vi "pRACTICA_1Y2_Punto_2_4.vi"() -> ()   [LabVIEW 2020]
panel:
  in  "Enum":T1(ring)
  out "?":string="La division es:"
  out "?":dbl
  in  "Numero 2":dbl
  in  "Numero 1":dbl
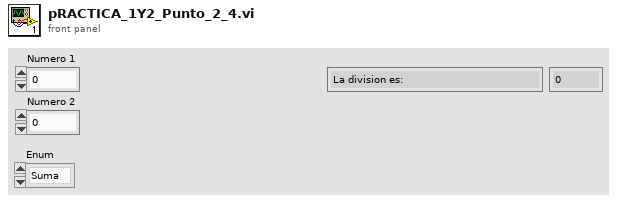
[diagram p1: front panel]
types:
  T1 = enum16{"Suma", "Resta", "Multiplicacion", "Division"}
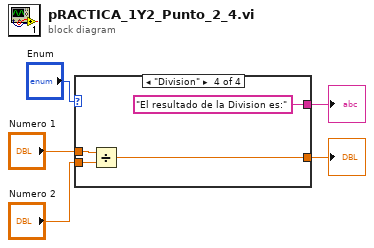
[diagram p0: block diagram]
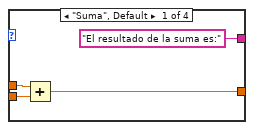
[diagram p2: hidden frame]
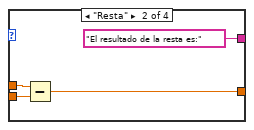
[diagram p3: hidden frame]
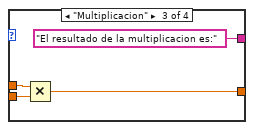
[diagram p4: hidden frame]
diagram:
  n1 = case shown="\"Division\"" "Enum" {
    tunnel: "Numero 1" -> [w9 w13 w16 w19]
    tunnel: "Numero 2" -> [w8 w12 w17 w20]
    tunnel: [w7 w11 w15 w18] -> w2
    tunnel: ["El resultado de la suma es:" "El resultado de la resta es:" "El resultado de la multiplicacion es:" "El resultado de la Division es:"] -> w1
    frame "Suma", Default {
      n2 = Add(x=w9, y=w8) -> (x+y=w7:dbl)
    }
    frame "Resta" {
      n3 = Subtract(x=w13, y=w12) -> (x-y=w11:dbl)
    }
    frame "Multiplicacion" {
      n4 = Multiply(x=w16, y=w17) -> (x*y=w15:dbl)
    }
    frame "Division" {
      n5 = Divide(x=w19, y=w20) -> (x/y=w18:dbl)
    }
  }
  "?" <- w2
  "?" <- w1
